vi "Read Binary Configuration.vi"(7 "Type":T1, 8 "error in (no error)":errorcluster, 9 "Default If Not Found":variant, 10 "Name":string, 11 "TransientConfiguration in":refnum<class "TransientConfiguration.lvclass">) -> (0 "error out":errorcluster, 1 "Not Found?":bool, 2 "Value":variant, 3 "TransientConfiguration out":refnum<class "TransientConfiguration.lvclass">)   [LabVIEW 2020, in "TransientConfiguration.lvclass"]
uses:
  <vilib>/gpm_packages/@cs/Configuration/Source/TransientConfiguration/TransientConfiguration.lvclass
  <vilib>/Utility/Data Type/Type Definitions/Data Type.ctl
  <vilib>/gpm_packages/@cs/Configuration/Source/TransientConfiguration/TransientConfiguration.lvclass/TransientConfiguration.ctl
  <vilib>/Utility/Data Type/NI_Data Type.lvlib
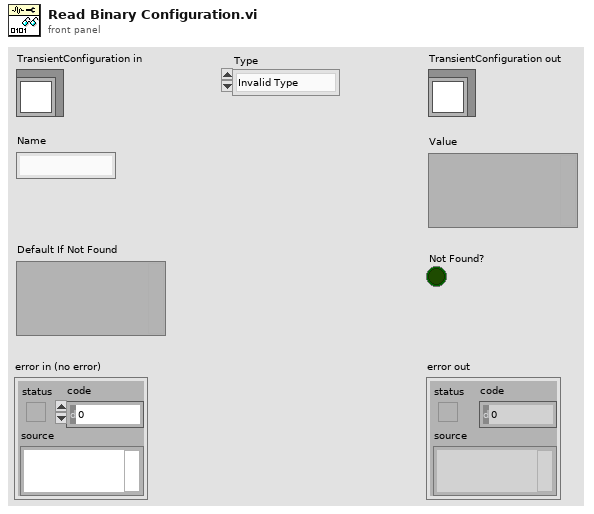
[diagram p1: front panel]
types:
  T1 = typedef "NI_Data Type.lvlib/Data Type.ctl" = enum8{"Invalid Type", "Void", "I8", "I16", "I32", "I64", "U8", "U16", "U32", "U64", "Single Float", "Double Float", "Extended Float", "Single Complex", "Double Complex", "Extended Complex", "Enum U8", "Enum U16", "Enum U32", "Enum U64", "Single Float With Unit", "Double Float With Unit", "Extended Float With Unit", "Single Complex with Unit", "Double Complex with Unit", "Extended Complex with Unit", "Boolean", "String", "Path", "Picture", "Tag", "Array", "Cluster", "Variant", "LV Variant", "Waveform", "Timestamp", "Digital Waveform", "Digital Data", "ExpressData", "Refnum", "External Data", "VI", "Poly VI", "LabVIEW Class Instance", "Fixed Point", "Set Collection", "Map Collection"}
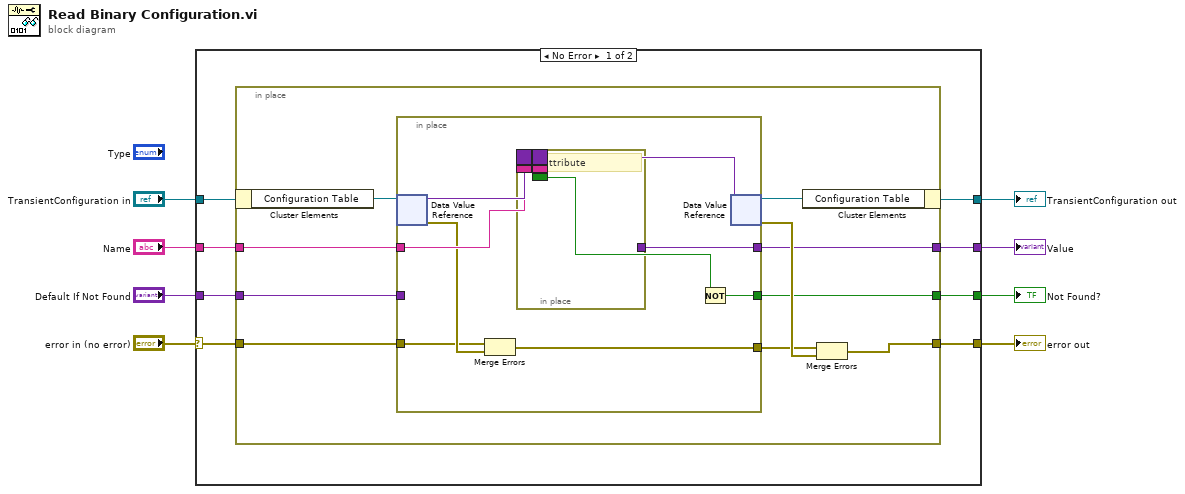
[diagram p0: block diagram]
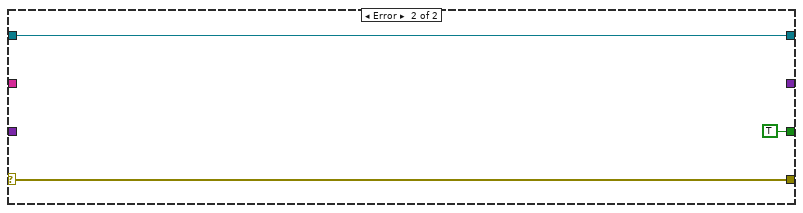
[diagram p2: hidden frame]
diagram:
  n1 = case shown="No Error" "error in (no error)" {
    selector: "error in (no error)" -> [w11 w39]
    tunnel: "TransientConfiguration in" -> [w16 w38]
    tunnel: [w15 w38] -> w7
    tunnel: "Name" -> [w14 _]
    tunnel: "Default If Not Found" -> [w13 _]
    tunnel: [w12 w39] -> w6
    tunnel: [w10 TRUE] -> w2
    tunnel: [w9 _] -> w1
    frame No Error {
      n2 = in-place {
        in-place-border: w14 -> [w24]
        in-place-border: w13 -> [w23]
        in-place-border: [w20] -> w12
        in-place-border: w11 -> [w19]
        in-place-border: [w18] -> w10
        in-place-border: [w17] -> w9
        n3 = in-place-cluster #1(w16) -> ("Configuration Table"=w26:refnum<data-value>)
        n4 = in-place {
          in-place-border: w24 -> [w34]
          in-place-border: w23 -> [_]
          in-place-border: [w31] -> w21
          in-place-border: w19 -> [w30]
          in-place-border: [w28] -> w18
          in-place-border: [w27] -> w17
          n5 = in-place-dvr #2(w26) -> (w35:variant, w32:errorcluster)
          n6 = Merge Errors(w30, w32) -> (w31:errorcluster)
          n7 = in-place {
            border: w35 -> [_]
            border: w34 -> [_]
            border: [_] -> w33
            border: _ -> [_]
            border: [_] -> w29
            in-place-border: [w36] -> w27
            # "Get attribute"
          }
          n8 = Not(x=w29) -> (.not. x?=w28:bool)
          n9 = in-place-dvr #2(w33) -> (w25:refnum<data-value>, w22:errorcluster)
        }
        n10 = in-place-cluster #1("Configuration Table"=w25) -> (w15:refnum<class "TransientConfiguration.lvclass">)
        n11 = Merge Errors(w21, w22) -> (w20:errorcluster)
      }
    }
    frame Error {
    }
  }
  "error out" <- w6
  "TransientConfiguration out" <- w7
  "Value" <- w1
  "Not Found?" <- w2
